vi "Initialise.vi"() -> (3 "Core Data out":T1)   [LabVIEW 2020, in "Amnesia.lvlib"]
uses:
  Amnesia.lvlib
  Scene/Scene.lvclass
  Graphics/Libraries/Raster/Rectangle Dimensions.ctl
  Graphics/Libraries/Raster/Raster.lvlib
  Core Data.ctl
  Scene/Mouse Button Held.ctl
  Graphics/Libraries/3D/3D.lvlib
  Graphics/Libraries/3D/Vector 3D.ctl
  Graphics/Libraries/3D/Transform.ctl
  <vilib>/Dataflow_G/G-Audio/G-Audio.lvlib
  <vilib>/Dataflow_G/G-Audio/Controls/Audio Device Format.ctl
  <vilib>/Dataflow_G/G-Audio/Controls/Audio Device Config.ctl
  fd7acbb8-dcf3-4e79-ae43-dfed6fdc6957.vi
  0dd0a49c-cf00-44f3-b489-91d0a4cbb1e5.vi
  <vilib>/Dataflow_G/G-Audio/Controls/Audio Device Refnum.ctl
  <vilib>/Dataflow_G/G-Audio/Audio Files/Polymorphic VIs/Open Audio File Read (Path).vi
  <vilib>/Dataflow_G/G-Audio/Audio Files/Polymorphic VIs/Get Audio File Info (Path).vi
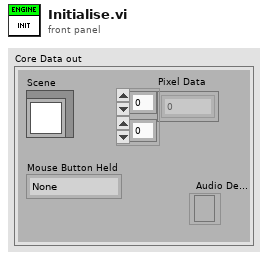
[diagram p1: front panel]
types:
  T1 = typedef "Amnesia.lvlib/Core Data.ctl" = cluster{"Pixel Data":u32[][], "Scene":refnum<class "Scene.lvclass">, "Mouse Button Held":T2, "Audio Device":T3}
  T2 = typedef "Scene.lvclass/Mouse Button Held.ctl" = enum16{"None", "Left", "Middle", "Right"}
  T3 = typedef "G-Audio.lvlib/Audio Device Refnum.ctl" = refnum<file>
  T4 = typedef "3D.lvlib/Transform.ctl" = cluster{"Position":T5, "Rotation":T5, "Scale":T5}
  T5 = typedef "3D.lvlib/Vector 3D.ctl" = cluster{"x":sgl, "y":sgl, "z":sgl}
  T6 = typedef "Raster.lvlib/Rectangle Dimensions.ctl" = cluster{"Width":u32, "Height":u32}
  T7 = typedef "G-Audio.lvlib/Audio Device Config.ctl" = cluster{"Sample Rate (Hz)":u32, "Channels":u32, "Format":T8}
  T8 = typedef "G-Audio.lvlib/Audio Device Format.ctl" = enum16{"Native", "U8", "I16", "I32", "SGL"}
  T9 = enum32{"invalid app kind", "Development System", "Run Time System", "Student Edition", "Embedded LabVIEW", "Evaluation", "Custom"}
  T10 = typedef "G-Audio.lvlib/Audio File Refnum.ctl" = refnum<file>
  T11 = typedef "3D.lvlib/Object.ctl" = cluster{"Triangles":T12[], "Transform":T4, "Name":string, "Alpha Blending Enabled":bool, "Alpha":dbl, "Turntable Enabled":bool, "Material":T15}
  T12 = typedef "3D.lvlib/Triangle.ctl" = cluster{"Vertex 1":T13, "Vertex 2":T13, "Vertex 3":T13, "Alpha":dbl, "Alpha Blending Enabled":bool, "Colour":u32, "Material":T15}
  T13 = typedef "3D.lvlib/Vertex.ctl" = cluster{"Position":T5, "UV":T14, "Colour":u32}
  T14 = typedef "Raster.lvlib/UV.ctl" = cluster{"u":sgl, "v":sgl}
  T15 = typedef "3D.lvlib/Material.ctl" = cluster{"Diffuse Colour":u32, "Texture":T16}
  T16 = typedef "Raster.lvlib/Texture.ctl" = cluster{"Pixels":refnum<data-value>, "Size":T6}
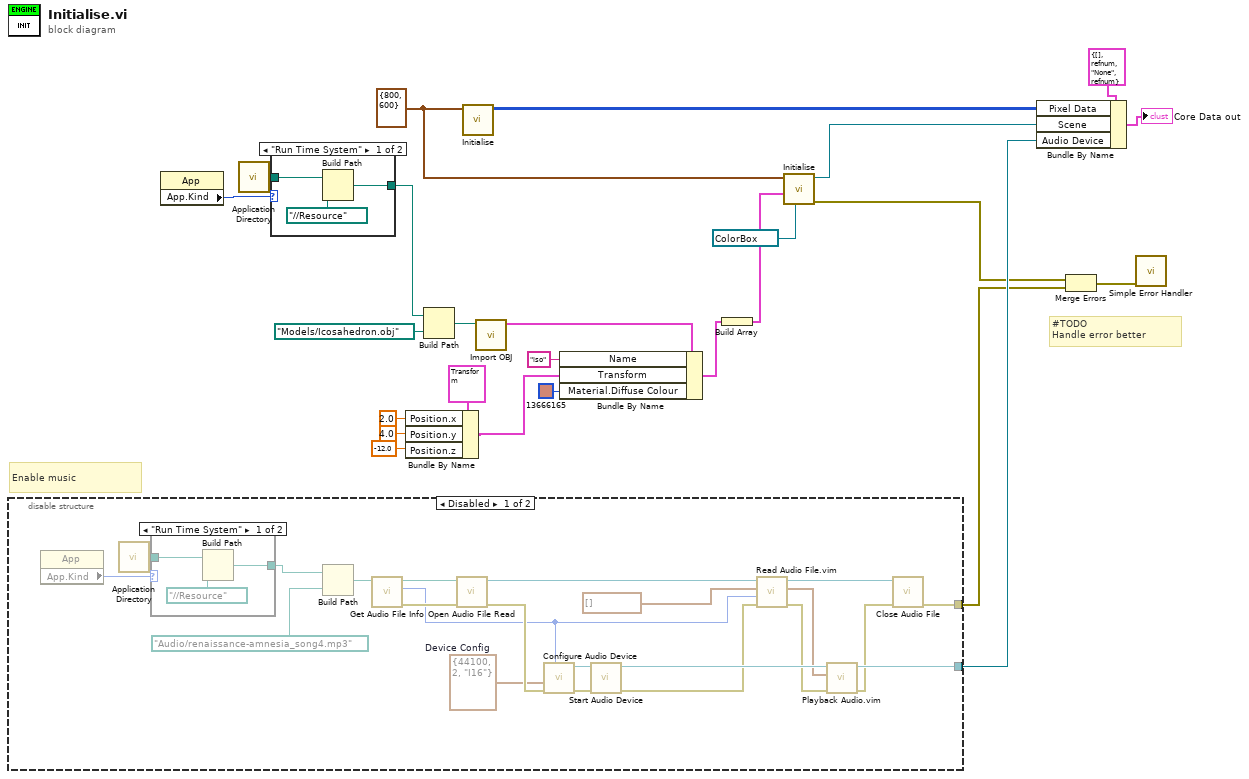
[diagram p0: block diagram]
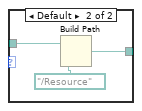
[diagram p2: hidden frame]
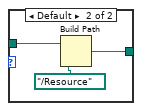
[diagram p4: hidden frame]
diagram:
  w20 = T6 {"Width"=800, "Height"=600} ("Screen Dimensions")
  # "Enable music"
  # "#TODO\nHandle error better"
  n1 = disable-structure shown="Disabled" {
    disable-tunnel: [w47 _] -> w5
    disable-tunnel: [w46 _] -> w3
    frame Disabled {
      w39 = T7 {"Sample Rate (Hz)"=44100, "Channels"=2, "Format"=enum."I16"}  # Device Config
      n2 = property class="App"() -> ("App.Kind"=w35:T9)  [unwired: 2 in, 2 out]
      n3 = call <vilib>:"Application Directory.vi"() -> ("Application Directory"=w36:path)
      n4 = case shown="\"Run Time System\"" w35 {
        tunnel: [w50 w53] -> w34
        tunnel: w36 -> [w48 w51]
        frame "Run Time System" {
          n5 = Build Path(base path=w48, name or relative path=path "../../Resource") -> (appended path=w50:path)
        }
        frame Default {
          n6 = Build Path(base path=w51, name or relative path=path "../Resource") -> (appended path=w53:path)
        }
      }
      n7 = Build Path(base path=w34, name or relative path=path "Audio/renaissance-amnesia_song4.mp3") -> (appended path=w32:path)
      n8 = call-poly <vilib>:"Get Audio File Info.vi"("Path In"=w32) -> ("error out"=w45:errorcluster, "PCM Frame Length"=w29:u64, "Path Out"=w38:path)  [unwired: 6 in, 2 out]
      n9 = call-poly <vilib>:"Open Audio File Read.vi"("error in (no error)"=w45, "Path"=w38) -> ("error out"=w40:errorcluster, "Audio File Refnum"=w28:T10)  [unwired: 8 in]
      n10 = call <vilib>:"Configure Audio Device.vi"("Buffer Size (4096)"=w29, "error in (no error)"=w40, "Device Config"=w39) -> ("error out"=w42:errorcluster, "Audio Device Refnum"=w41:T3)  [unwired: 5 in, 2 out]
      n11 = call <vilib>:"Start Audio Device.vi"("error in (no error)"=w42, "Audio Device Refnum In"=w41) -> ("error out"=w43:errorcluster, "Audio Device Refnum Out"=w44:T3)  [unwired: 8 in]
      n12 = call "Read Audio File.vim"("error in (no error)"=w43, "Frames To Read"=w29, "Data Format"=waveform(i16)[] [], "Audio File Refnum In"=w28) -> ("error out"=w31:errorcluster, "Audio Data"=w30:waveform(i16)[], "Audio File Refnum Out"=w27:T10)  [unwired: 3 in, 2 out]
      n13 = call "Playback Audio.vim"("error in (no error)"=w31, "Audio Data"=w30, "Audio Device Refnum In"=w44) -> ("error out"=w26:errorcluster, "Audio Device Refnum Out"=w47:T3)  [unwired: 7 in]
      n14 = call <vilib>:"Close Audio File.vi"("error in (no error)"=w26, "Audio File Refnum In"=w27) -> ("error out"=w46:errorcluster)  [unwired: 9 in]
    }
    frame Enabled {
    }
  }
  n15 = property class="App"() -> ("App.Kind"=w22:T9)  [unwired: 2 in, 2 out]
  n16 = call <vilib>:"Application Directory.vi"() -> ("Application Directory"=w21:path)
  n17 = case shown="\"Run Time System\"" w22 {
    tunnel: [w56 w59] -> w17
    tunnel: w21 -> [w54 w57]
    frame "Run Time System" {
      n18 = Build Path(base path=w54, name or relative path=path "../../Resource") -> (appended path=w56:path)
    }
    frame Default {
      n19 = Build Path(base path=w57, name or relative path=path "../Resource") -> (appended path=w59:path)
    }
  }
  n20 = Bundle By Name(cluster=T4 {"Position"={"x"=2.0, "y"=1.0, "z"=-5.0}, "Rotation"={"x"=0.0, "y"=0.0, "z"=0.0}, "Scale"={"x"=0.0, "y"=0.0, "z"=0.0}} ("Transform"), "Position.x"=sgl 2.0, "Position.y"=sgl 4.0, "Position.z"=sgl -12.0) -> (w8:T4)
  n21 = Build Path(base path=w17, name or relative path=path "Models/Icosahedron.obj") -> (appended path=w16:path)
  n22 = call "Initialise.vi"("Screen Dimensions"=w20) -> ("Pixel Data out"=w23:u32[][])  [unwired: 10 in]
  n23 = call "Import OBJ.vi"("Object"=w16) -> ("Object"=w14:T11)  [unwired: 9 in, 1 out]
  n24 = Bundle By Name(cluster=w14, "Name"="iso", "Transform"=w8, "Material.Diffuse Colour"=u32 13666165) -> (w13:T11)
  n25 = Build Array(w13) -> (w18:T11[])
  n26 = call "Initialise.vi"("Diffuse Colour"=refnum<vi> refnum, "Objects"=w18, "Screen Dimensions"=w20) -> ("error out"=w4:errorcluster, "Scene out"=w19:refnum<class "Scene.lvclass">)  [unwired: 7 in]
  n27 = Bundle By Name(cluster=T1 {"Pixel Data"=[], "Scene"=refnum, "Mouse Button Held"=enum."None", "Audio Device"=refnum} ("Core Data"), "Pixel Data"=w23, "Scene"=w19, "Audio Device"=w5) -> (→"Core Data out":T1)
  n28 = Merge Errors(w4, w3) -> (w2:errorcluster)
  n29 = call <vilib>:"Simple Error Handler.vi"("error in (no error)"=w2) -> ()  [unwired: 4 in, 5 out]
